vi "Timeout Watchdog.vi"(11 "Buffered Log Sink in":refnum<class "Buffered Log Sink.lvclass">) -> ()   [LabVIEW 2019, in "Buffered Log Sink.lvclass"]
uses:
  <vilib>/gpm_packages/@cs/event-logger/Source/Buffered Log Sink/Buffered Log Sink.lvclass
  <vilib>/gpm_packages/@cs/event-logger/Source/Buffered Log Sink/Buffered Log Sink.lvclass/Buffered Log Sink.ctl
  <vilib>/gpm_packages/@cs/event-logger/Source/Composed Log/Log Sink/Log Sink.lvclass
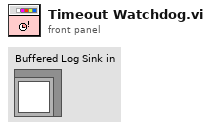
[diagram p1: front panel]
types:
  T1 = typedef "Composed Log.lvlib/Log Packet.ctl" = cluster{"Data To Log":string, "Source":string, "Event Level":T2, "Event Time":timestamp}
  T2 = typedef "Composed Log.lvlib/Log Level.ctl" = enum16{"Debug", "Info", "Warning", "Error", "Critical"}
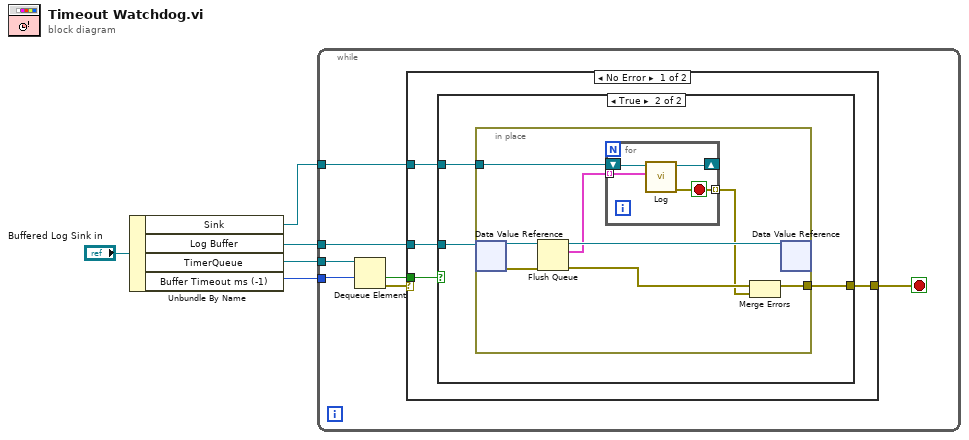
[diagram p0: block diagram]
diagram:
  n1 = Unbundle By Name("Buffered Log Sink in") -> ("Sink"=w1:refnum<class "Log Sink.lvclass">, "Log Buffer"=w4:refnum<data-value>, "TimerQueue"=w3:refnum<queue>, "Buffer Timeout ms (-1)"=w2:i32)
  n2 = while {
    tunnel: w4 -> [w8]
    tunnel: w3 -> [w12]
    tunnel: w2 -> [w11]
    tunnel: w1 -> [w7]
    stop <- w6 stop-if-true
    n3 = Dequeue Element(queue=w12, timeout in ms (-1)=w11) -> (timed out?=w9:bool, error out=w10:errorcluster)  [unwired: 1 in, 2 out]
    n4 = case shown="No Error" w10 {
      selector: w10 -> [_ w32]
      tunnel: w9 -> [w16 _]
      tunnel: w8 -> [w15 _]
      tunnel: w7 -> [w14 _]
      tunnel: [w13 w32] -> w6
      frame No Error {
        n5 = case shown="True" w16 {
          tunnel: w15 -> [_ w19]
          tunnel: w14 -> [_ w17]
          tunnel: [_ w18] -> w13
          frame False {
          }
          frame True {
            n6 = in-place {
              in-place-border: [w21] -> w18
              in-place-border: w17 -> [w23]
              n7 = in-place-dvr #1(w19) -> (w27:refnum<queue>, w26:errorcluster)
              n8 = Flush Queue(queue=w27, error in (no error)=w26) -> (queue out=w24:refnum<queue>, remaining elements=w22:T1[], error out=w25:errorcluster)
              n9 = for {
                shift-right: [w29] -> _
                shift-left: w23 -> [w31]
                tunnel: w22 -> [w30] mode=indexing
                tunnel: [w28] -> w20 mode=indexing
                stop <- w28 stop-if-true
                n10 = call-dynamic "Log.vi"("Log Packet"=w30, "Log Sink in"=w31) -> ("error out"=w28:errorcluster, "Log Sink out"=w29:refnum<class "Log Sink.lvclass">)  [unwired: 8 in]
              }
              n11 = Merge Errors(w25, w20) -> (w21:errorcluster)
              n12 = in-place-dvr #1(w24) -> ()  [unwired: 2 out]
            }
          }
        }
      }
      frame Error {
      }
    }
  }
